vi "getCamerasPositionByID.vi"(9 "cameras id":dbl[](array[numeric]), 11 "Field Size 2":T1) -> (3 "Cameras Positions":dbl[][](array[numeric]))   [LabVIEW 2021]
uses:
  399b7754-30dd-4449-a6a8-6758c9e68e52.vi
  <vilib>/Array/Sort 2D Array - Pop Stack.vi
  <vilib>/Array/Sort 2D Array - Push Stack.vi
  399b7754-30dd-4449-a6a8-6758c9e68e52.vi/269d4b3b-47f5-49e3-8884-44851e4dd9d5.vi
  399b7754-30dd-4449-a6a8-6758c9e68e52.vi/6d99389c-673d-4efb-bf33-19b32bcf4cf8.vi
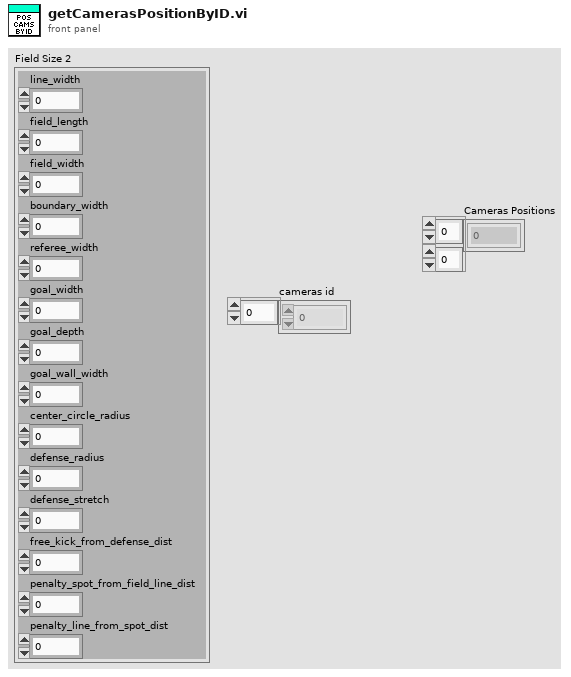
[diagram p1: front panel]
types:
  T1 = cluster{"line_width":u32, "field_length":u32, "field_width":u32, "boundary_width":u32, "referee_width":u32, "goal_width":u32, "goal_depth":u32, "goal_wall_width":u32, "center_circle_radius":u32, "defense_radius":u32, "defense_stretch":u32, "free_kick_from_defense_dist":u32, "penalty_spot_from_field_line_dist":u32, "penalty_line_from_spot_dist":u32}
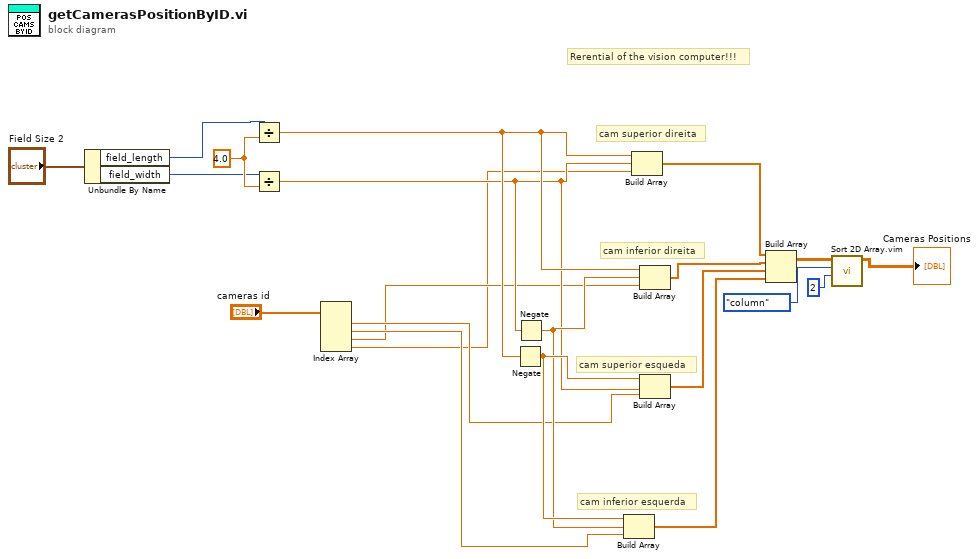
[diagram p0: block diagram]
diagram:
  w20 = 4.0 ("y")
  # "Rerential of the vision computer!!!"
  # "cam inferior esquerda"
  # "cam superior esqueda"
  # "cam inferior direita"
  # "cam superior direita"
  n1 = Unbundle By Name("Field Size 2") -> ("field_length"=w19:u32, "field_width"=w18:u32)
  n2 = Divide(x=w19, y=w20) -> (x/y=w8:dbl)
  n3 = Divide(x=w18, y=w20) -> (x/y=w7:dbl)
  n4 = Index Array(array="cameras id") -> (element #1=w4:dbl, element #2=w3:dbl, element #3=w2:dbl, element #4=w1:dbl)  [unwired: 4 in]
  n5 = Negate(x=w8) -> (-x=w17:dbl)
  n6 = Negate(x=w7) -> (-x=w16:dbl)
  n7 = Build Array(w17, w16, w3) -> (w9:dbl[])
  n8 = Build Array(w8, w7, w1) -> (w12:dbl[])
  n9 = Build Array(w8, w16, w2) -> (w11:dbl[])
  n10 = Build Array(w17, w7, w4) -> (w10:dbl[])
  n11 = Build Array(w12, w11, w10, w9) -> (w15:dbl[][])
  n12 = call "Sort 2D Array.vim"("index"=2, "dimension to index (column)"=enum16{"column", "row"}."column", "2D array"=w15) -> ("sorted 2D array"=→"Cameras Positions":dbl[][])  [unwired: 7 in, 1 out]
